vi "Initialize.vi"(8 "error in":errorcluster, 10 "SubPanel init":T1, 11 "SubPanel in":refnum<class "xceSubPanel.lvclass">) -> (0 "error out":errorcluster, 3 "SubPanel out":refnum<class "xceSubPanel.lvclass">)   [LabVIEW 2013, in "xceSubPanel.lvclass"]
doc: "Sets the information need for the SubPanel class to operate."
uses:
  xceSubPanel.lvclass
  SubPanel init.ctl
  <vilib>/NI/AMC/Message Queue.ctl
  <vilib>/NI/AMC/Message.ctl
  <vilib>/NI/Tools/Keyed Array/KeyedArray.ctl
  xceSubPanel.lvclass/xceSubPanel.ctl
  <vilib>/NI/AMC/AMC.lvlib
  <vilib>/NI/Tools/Keyed Array/Tools_KeyedArray.lvlib
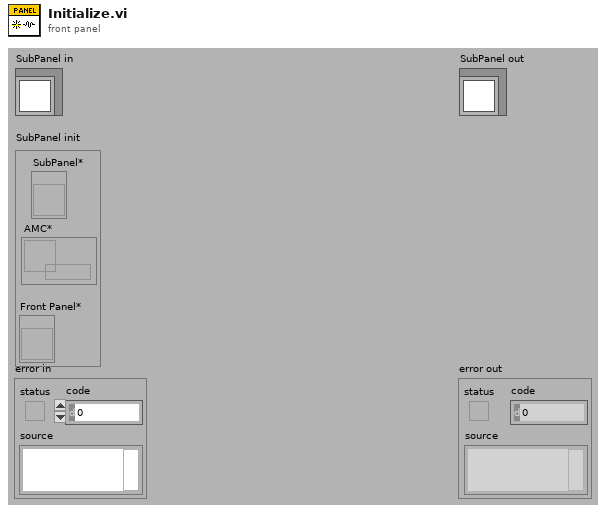
[diagram p1: front panel]
types:
  T1 = typedef "xceSubPanel.lvclass/SubPanel init.ctl" = cluster{"SubPanel*":refnum<vi>, "Front Panel*":refnum<vi>, "AMC*":T2}
  T2 = typedef "AMC.lvlib/Message Queue.ctl" = refnum<queue>
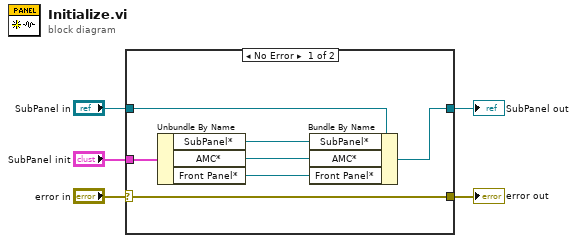
[diagram p0: block diagram]
diagram:
  n1 = case shown="No Error" "error in" {
    selector: "error in" -> [w12 w14]
    tunnel: [w12 w14] -> w4
    tunnel: [w8 w13] -> w2
    tunnel: "SubPanel in" -> [w9 w13]
    tunnel: "SubPanel init" -> [w11 _]
    frame No Error {
      n2 = Unbundle By Name(w11) -> ("SubPanel*"=w10:refnum<vi>, "AMC*"=w6:T2, "Front Panel*"=w7:refnum<vi>)
      n3 = Bundle By Name(cluster=w9, "SubPanel*"=w10, "AMC*"=w6, "Front Panel*"=w7) -> (w8:refnum<class "xceSubPanel.lvclass">)
    }
    frame Error {
    }
  }
  "error out" <- w4
  "SubPanel out" <- w2
